vi "MainPane Slide.vi"(8 "error in (no error)":errorcluster, 9 "Slide Direction":T1=enum."Back", 10 "Enqueuer":refnum<class "Message Enqueuer.lvclass">, 11 "MainController in":refnum<class "MainController.lvclass">) -> (0 "error out":errorcluster, 3 "MainController out":refnum<class "MainController.lvclass">)   [LabVIEW 2012, in "Win8uiFramework.lvlib" / "MainController.lvclass"]
uses:
  MainController.lvclass
  <vilib>/ActorFramework/Message Enqueuer/Message Enqueuer.lvclass
  Slide Direction.ctl
  <vilib>/Utility/miscctls.llb/LVPointTypeDef.ctl
  MainController.lvclass/MainController.ctl
  Insert Into SubPanel Msg.lvclass/Insert Into SubPanel Msg.ctl
  <vilib>/ActorFramework/Message Enqueuer/Message Enqueuer.lvclass/Message Enqueuer.ctl
  Read Active SubPanel.vi
  Read Inactive SubPanel.vi
  Read Main Pane.vi
  Read MainPane Enqueuer.vi
  Write Active SubPanel.vi
  Write Inactive SubPanel.vi
  Write MainPane Enqueuer.vi
  <vilib>/ActorFramework/Message Enqueuer/Enqueue.vi
  <vilib>/ActorFramework/Message Priority Queue/Priority Enqueue.vi
  <vilib>/Utility/error.llb/Simple Error Handler.vi
  Insert Into SubPanel Msg.lvclass
  <vilib>/ActorFramework/Stop Msg/Stop Msg.lvclass
  Remove From SubPanel Msg.lvclass
  Win8uiFramework.lvlib
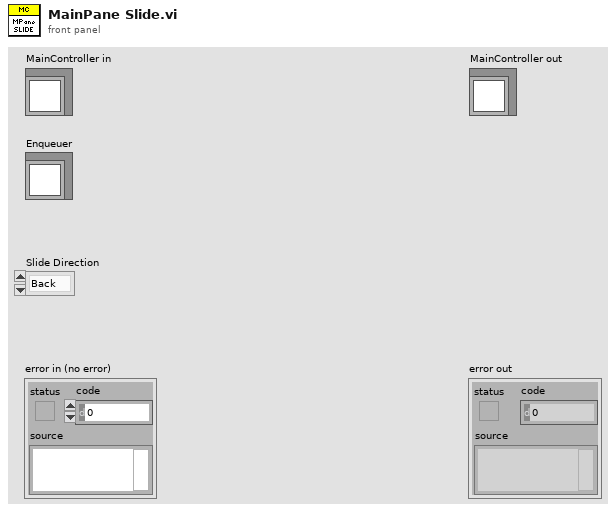
[diagram p1: front panel]
types:
  T1 = typedef "Win8uiFramework.lvlib/Slide Direction.ctl" = enum16{"Forwards", "Back"}
  T2 = typedef "LVPointTypeDef.ctl" = cluster{"Horizontal":i16, "Vertical":i16}
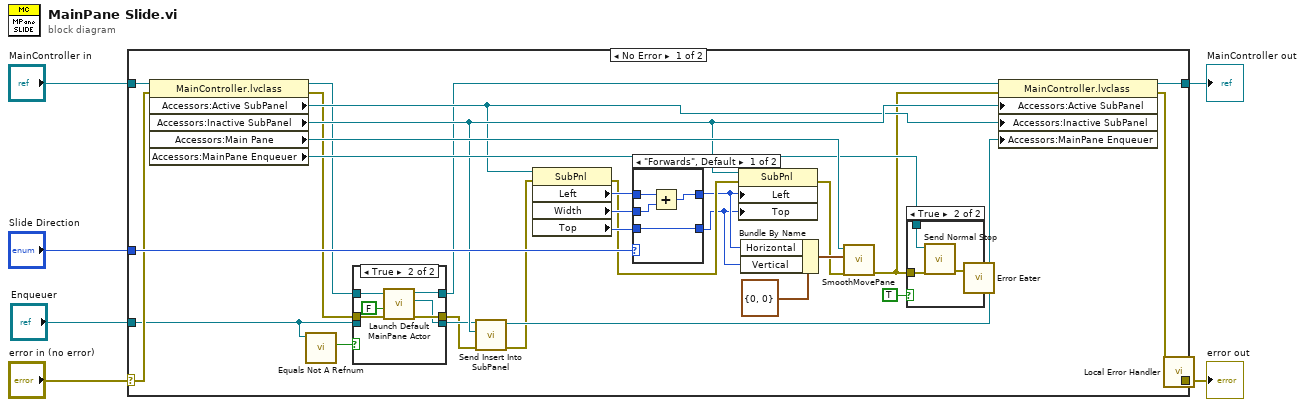
[diagram p0: block diagram]
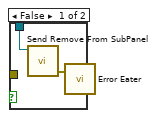
[diagram p3: hidden frame]
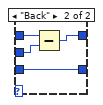
[diagram p4: hidden frame]
diagram:
  n1 = case shown="No Error" "error in (no error)" {
    selector: "error in (no error)" -> [w31 w60]
    tunnel: [w9 w60] -> w5
    tunnel: [w22 w59] -> w3
    tunnel: "MainController in" -> [w36 w59]
    tunnel: "Enqueuer" -> [w17 _]
    tunnel: "Slide Direction" -> [w35 _]
    frame No Error {
      n2 = property class="MainController.lvclass"(reference=w36, error in=w31) -> (reference out=w14:refnum<class "MainController.lvclass">, error out=w15:errorcluster, "Accessors:Active SubPanel"=w20:refnum<vi>, "Accessors:Inactive SubPanel"=w21:refnum<vi>, "Accessors:Main Pane"=w26:refnum<vi>, "Accessors:MainPane Enqueuer"=w23:refnum<class "Message Enqueuer.lvclass">)
      n3 = call <vilib>:"Equals Not A Refnum.vi"("Message Enqueuer"=w17) -> ("Not a refnum?"=w18:bool)  [unwired: 10 in]
      n4 = case shown="True" w18 {
        tunnel: w17 -> [w39 _]
        tunnel: [w39 w41] -> w16
        tunnel: w14 -> [w38 w45]
        tunnel: w15 -> [w37 w43]
        tunnel: [w38 w44] -> w13
        tunnel: [w37 w42] -> w12
        frame False {
        }
        frame True {
          n5 = call-dynamic "Launch Default MainPane Actor.vi"("error in (no error)"=w43, "Stop Existing? (T)"=FALSE, "MainController in"=w45) -> ("error out"=w42:errorcluster, "Enqueuer"=w41:refnum<class "Message Enqueuer.lvclass">, "MainController out"=w44:refnum<class "MainController.lvclass">)  [unwired: 6 in]
        }
      }
      n6 = call "Send Insert Into SubPanel.vi"("error in (no error)"=w12, "SubPanel Ref"=w21, "Message Enqueuer"=w16) -> ("error out"=w11:errorcluster, "Message Enqueuer out"=w19:refnum<class "Message Enqueuer.lvclass">)  [unwired: 7 in]
      n7 = property class="SubPnl"(reference=w20, error in=w11) -> (error out=w30:errorcluster, "Left"=w34:i32, "Width"=w33:u32, "Top"=w32:i32)  [unwired: 1 out]
      n8 = case shown="\"Forwards\", Default" w35 {
        tunnel: w34 -> [w54 w58]
        tunnel: w33 -> [w53 w57]
        tunnel: [w52 w56] -> w28
        tunnel: w32 -> [w51 w55]
        tunnel: [w51 w55] -> w27
        frame "Forwards", Default {
          n9 = Add(x=w54, y=w53) -> (x+y=w52:u32)
        }
        frame "Back" {
          n10 = Subtract(x=w58, y=w57) -> (x-y=w56:u32)
        }
      }
      n11 = property class="SubPnl"(reference=w21, error in=w30, "Left"=w28, "Top"=w27) -> (error out=w24:errorcluster)  [unwired: 1 out]
      n12 = Bundle By Name(cluster=T2 {"Horizontal"=0, "Vertical"=0} ("Origin"), "Horizontal"=w28, "Vertical"=w27) -> (w25:T2)
      n13 = call "SmoothMovePane.vi"("error in (no error)"=w24, "Origin"=w25, "Pane in"=w26) -> ("error out"=w8:errorcluster)  [unwired: 8 in]
      n14 = case shown="True" TRUE {
        tunnel: w23 -> [w47 w50]
        tunnel: w8 -> [_ w48]
        frame False {
          n15 = call "Send Remove From SubPanel.vi"("Message Enqueuer"=w47) -> ("error out"=w46:errorcluster)  [unwired: 9 in, 1 out]
          n16 = call "Error Eater.vi"("error in (no error)"=w46) -> ()  [unwired: 2 in]
        }
        frame True {
          n17 = call <vilib>:"Send Normal Stop.vi"("error in (no error)"=w48, "Message Enqueuer"=w50) -> ("error out"=w49:errorcluster)  [unwired: 9 in]
          n18 = call "Error Eater.vi"("error in (no error)"=w49) -> ()  [unwired: 2 in]
        }
      }
      n19 = property class="MainController.lvclass"(reference=w13, error in=w8, "Accessors:Active SubPanel"=w21, "Accessors:Inactive SubPanel"=w20, "Accessors:MainPane Enqueuer"=w19) -> (reference out=w22:refnum<class "MainController.lvclass">, error out=w10:errorcluster)
      n20 = call "Local Error Handler.vi"("error in (no error)"=w10) -> ("error out"=w9:errorcluster)  [unwired: 18 in]
    }
    frame Error {
    }
  }
  "error out" <- w5
  "MainController out" <- w3
